vi "FTP.vi"(8 "error in (no error)":errorcluster caption="错误输入（无错误）", 10 "远程路径":string, 11 "local path":path caption="文件路径") -> (0 "error out":errorcluster caption="错误输出")   [LabVIEW 2020]
uses:
  <vilib>/FTP/NI_FTP.lvlib
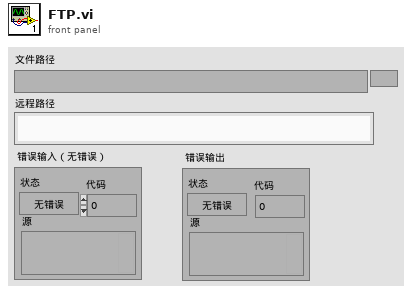
[diagram p1: front panel]
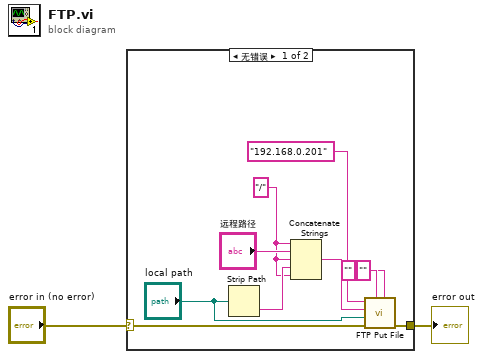
[diagram p0: block diagram]
diagram:
  n1 = case shown="无错误" "error in (no error)" {
    selector: "error in (no error)" -> [w7 w13]
    tunnel: [w8 w13] -> w2
    frame No Error {
      w6 = "/" ("字符串")
      n2 = Strip Path(path="local path") -> (name=w10:string)  [unwired: 1 out]
      n3 = Concatenate Strings(w6, "远程路径", w6, w10, w6) -> (w11:string)
      n4 = call <vilib>:"FTP Put File.vi"("password"="", "user"="", "error in (no error)"=w7, "local path"="local path", "remote path"=w11, "host"="192.168.0.201") -> ("error out"=w8:errorcluster)  [unwired: 4 in, 1 out]
    }
    frame Error {
    }
  }
  "error out" <- w2
